vi "UploadtoArduino.vi"(8 "Sketch.ino":string, 9 "path to sketch folder":path, 10 "serial port":string, 11 "path to bossac":path) -> (2 "standard error":string, 3 "standard output":string)   [LabVIEW 2019]
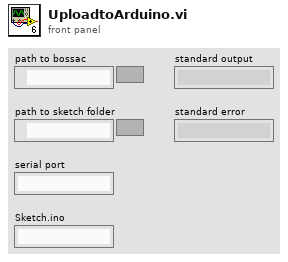
[diagram p1: front panel]
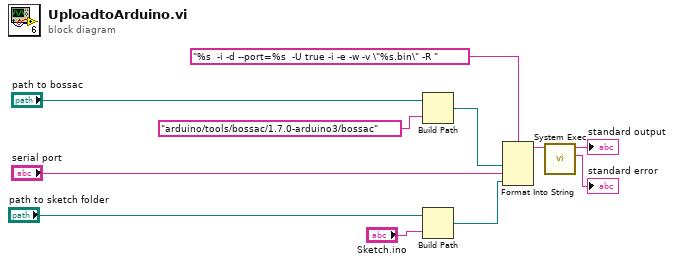
[diagram p0: block diagram]
diagram:
  n1 = Build Path(base path="path to bossac", name or relative path="arduino/tools/bossac/1.7.0-arduino3/bossac") -> (appended path=w1:path)
  n2 = Build Path(base path="path to sketch folder", name or relative path="Sketch.ino") -> (appended path=w4:path)
  n3 = Format Into String(format string="%s  -i -d --port=%s  -U true -i -e -w -v \"%s.bin\" -R ", w1, "serial port", w4) -> (resulting string=w2:string)  [unwired: 2 in, 1 out]
  n4 = call <vilib>:"System Exec.vi"("command line"=w2) -> ("standard error"=→"standard error":string, "standard output"=→"standard output":string)  [unwired: 7 in, 2 out]
